vi "Shooter.vi"(4 "FiringCylinder":T1={"DevStatus"={"status"=FALSE, "code"=0, "source"=""}, "Solenoid Module"=enum."Solenoid Module 1", "Forward Solenoid Channel"=enum."Invalid", "Reverse Solenoid Channel"=enum."Invalid"}, 6 "Kicker":T1={"DevStatus"={"status"=FALSE, "code"=0, "source"=""}, "Solenoid Module"=enum."Solenoid Module 1", "Forward Solenoid Channel"=enum."Invalid", "Reverse Solenoid Channel"=enum."Invalid"}, 7 "Action":T4=enum."Shoot", 8 "error in":errorcluster, 9 "Wait3":u32, 10 "Wait2":u32, 11 "Wait1":u32) -> (0 "error out":errorcluster)   [LabVIEW 2013]
doc: "Shooter has the following actions:\n-Init: takes a single solenoid reference for the kicker and firing cylinder and passes them onto the single solenoid VI.\n-Shoot:\n +Actuates the firing cylinders.\n +Waits a specified amount of time (Wait1).\n +Actuates the kicker.\n +Waits a specified amount of time (Wait2).\n +Retracts the kicker.\n +Waits a specified amount of time (Wait3).\n +Retracts the firing cylinders."
uses:
  ShooterAction.ctl
  <vilib>/Rock Robotics/WPI/Solenoid/WPI_SolenoidDevRef.ctl
  <vilib>/Rock Robotics/SystemInterfaces/Typedef/FPGA_TypedefSolenoidModule.ctl
  <vilib>/Rock Robotics/WPI/Solenoid/WPI_SolenoidChannel.ctl
  PnuematicMode.ctl
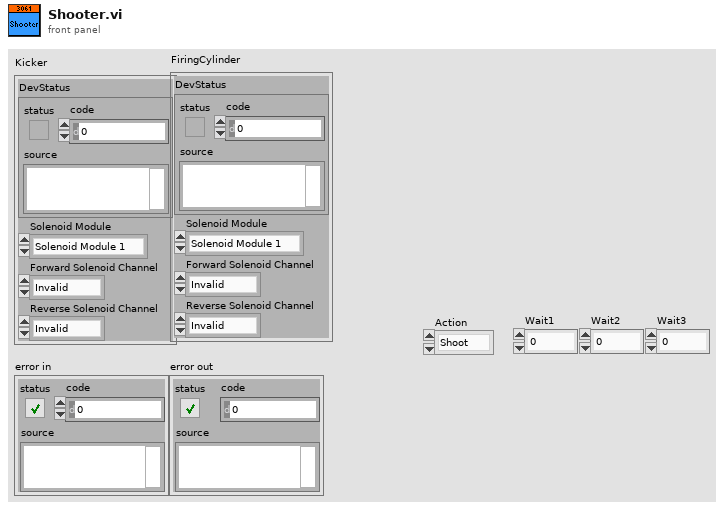
[diagram p1: front panel]
types:
  T1 = typedef "WPI_SolenoidDevRef.ctl" = cluster{"DevStatus":errorcluster, "Solenoid Module":T2, "Forward Solenoid Channel":T3, "Reverse Solenoid Channel":T3}
  T2 = typedef "FPGA_TypedefSolenoidModule.ctl" = enum16{"Solenoid Module 1", "Solenoid Module 2"}
  T3 = typedef "WPI_SolenoidChannel.ctl" = enum8{"Solenoid 1", "Solenoid 2", "Solenoid 3", "Solenoid 4", "Solenoid 5", "Solenoid 6", "Solenoid 7", "Solenoid 8", "Invalid"}
  T4 = typedef "ShooterAction.ctl" = enum16{"Init", "Shoot"}
  T5 = typedef "PnuematicMode.ctl" = enum16{"Init", "SetState", "Disable"}
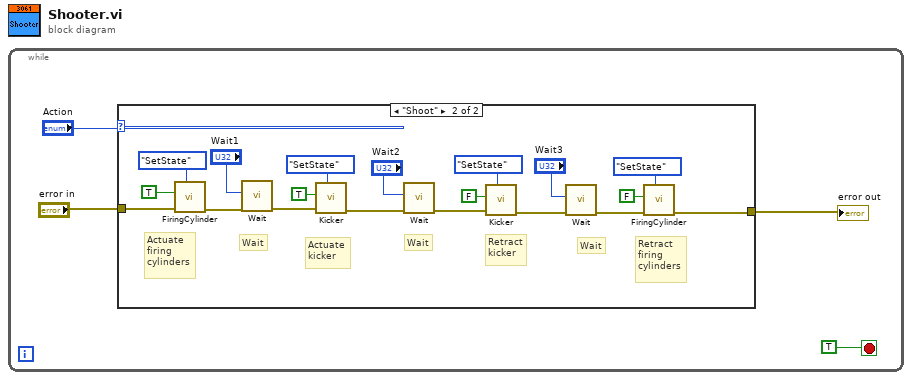
[diagram p0: block diagram]
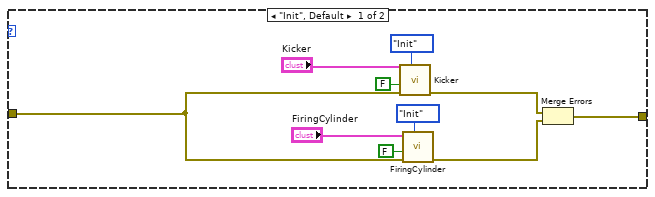
[diagram p2: hidden frame]
diagram:
  n1 = while {
    stop <- TRUE stop-if-true
    n2 = case shown="\"Shoot\"" "Action" {
      tunnel: "error in" -> [w8 w25]
      tunnel: [w5 w32] -> w1
      frame "Init", Default {
        n3 = call "Kicker.vi"("Mode"=PnuematicMode."Init", "error in (no error)"=w8, "Default Position"=FALSE, "SolenoidDevRef"="Kicker") -> ("error out"=w7:errorcluster)  [unwired: 7 in]
        n4 = call "FiringCylinder.vi"("Mode"=PnuematicMode."Init", "error in (no error)"=w8, "Default Position"=FALSE, "SolenoidDevRef"="FiringCylinder") -> ("error out"=w6:errorcluster)  [unwired: 7 in]
        n5 = Merge Errors(w7, w6) -> (w5:errorcluster)
      }
      frame "Shoot" {
        # "Retract\nfiring\ncylinders"
        # "Wait"
        # "Retract\nkicker"
        # "Wait"
        # "Actuate\nkicker"
        # "Wait"
        # "Actuate\nfiring\ncylinders"
        n6 = call "FiringCylinder.vi"("Mode"=PnuematicMode."SetState", "error in (no error)"=w25, "State"=TRUE) -> ("error out"=w24:errorcluster)  [unwired: 8 in]
        n7 = call "Wait.vi"("error in"=w24, "milliseconds to wait"="Wait1") -> ("error out"=w33:errorcluster)  [unwired: 9 in]
        n8 = call "Kicker.vi"("Mode"=PnuematicMode."SetState", "error in (no error)"=w33, "State"=TRUE) -> ("error out"=w30:errorcluster)  [unwired: 8 in]
        n9 = call "Wait.vi"("error in"=w30, "milliseconds to wait"="Wait2") -> ("error out"=w29:errorcluster)  [unwired: 9 in]
        n10 = call "Kicker.vi"("Mode"=PnuematicMode."SetState", "error in (no error)"=w29, "State"=FALSE) -> ("error out"=w28:errorcluster)  [unwired: 8 in]
        n11 = call "Wait.vi"("error in"=w28, "milliseconds to wait"="Wait3") -> ("error out"=w31:errorcluster)  [unwired: 9 in]
        n12 = call "FiringCylinder.vi"("Mode"=PnuematicMode."SetState", "error in (no error)"=w31, "State"=FALSE) -> ("error out"=w32:errorcluster)  [unwired: 8 in]
      }
    }
    "error out" <- w1
  }
